vi "配置读取写入.vi"(7 "write":bool, 8 "error in (no error)":errorcluster, 11 "配置":T1={"url"="http://data.watersystem.com.cn:50040", "loginTokenRequest"={"clientId"="wqms_equip", "clientSecret"="2gJxw%vZkRGX8K7Se$^q", "grantType"="password", "password"="123456", "scope"="read", "userName"="equipapi", "userType"="equip"}, "自动获取MN"=TRUE}) -> (0 "error out":errorcluster, 3 "配置输出":T1={"url"="http://dev.watersystem.com.cn:36091", "loginTokenRequest"={"clientId"="test_client", "clientSecret"="test_secret", "grantType"="password", "password"="59315200", "scope"="read", "userName"="STDTEST001", "userType"="equip"}, "自动获取MN"=TRUE})   [LabVIEW 2022 SP3, in "opSignIn.lvlib"]
uses:
  opSignIn.lvlib
  <vilib>/Utility/config.llb/NI_LVConfig.lvlib
  <userlib>/_OpenG.lib/variantconfig/variantconfig.llb/openg_variant_configuration_file.lvlib
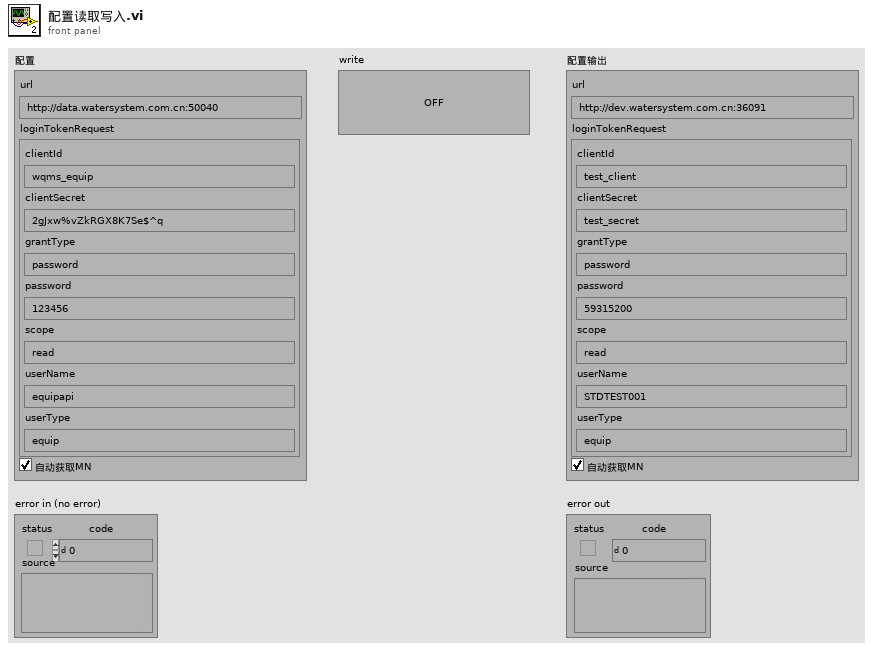
[diagram p1: front panel]
types:
  T1 = cluster{"url":string, "loginTokenRequest":cluster{"clientId":string, "clientSecret":string, "grantType":string, "password":string, "scope":string, "userName":string, "userType":string}, "自动获取MN":bool}
  T2 = typedef "NI_LVConfig.lvlib/Config Data RefNum.ctl" = refnum<k1>
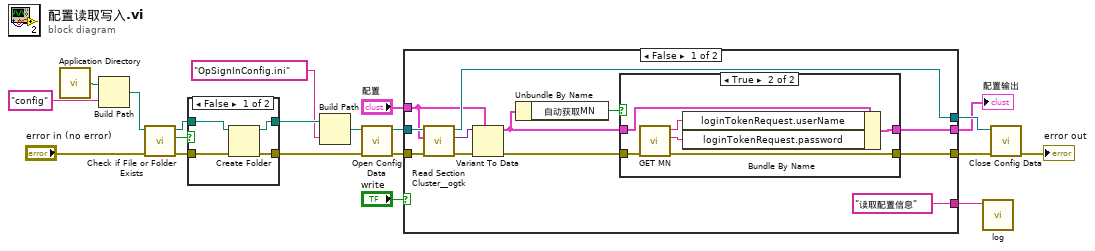
[diagram p0: block diagram]
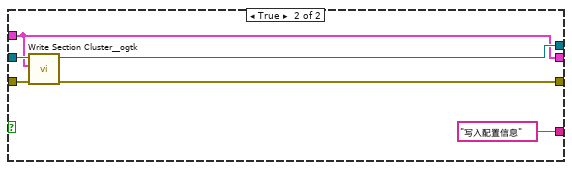
[diagram p3: hidden frame]
diagram:
  n1 = call <vilib>:"Application Directory.vi"() -> ("Application Directory"=w15:path)
  n2 = Build Path(base path=w15, name or relative path="config" ("名称或相对路径")) -> (appended path=w13:path)
  n3 = call <vilib>:"Check if File or Folder Exists.vi"("error in (no error)"="error in (no error)", "path"=w13) -> ("error out"=w10:errorcluster, "file or folder exists?"=w12:bool, "dup path"=w11:path)  [unwired: 7 in]
  n4 = case shown="False" w12 {
    tunnel: w11 -> [w24 w26]
    tunnel: [w23 w26] -> w9
    tunnel: w10 -> [w22 w25]
    tunnel: [w21 w25] -> w3
    frame False {
      n5 = Create Folder(path (use dialog)=w24, error in=w22) -> (created path=w23:path, error out=w21:errorcluster)  [unwired: 1 in, 1 out]
    }
    frame True {
    }
  }
  n6 = Build Path(base path=w9, name or relative path="OpSignInConfig.ini" ("名称或相对路径")) -> (appended path=w8:path)
  n7 = call <vilib>:"Open Config Data.vi"("error in (no error)"=w3, "configuration file path"=w8) -> ("error out"=w18:errorcluster, "refnum"=w20:T2)  [unwired: 7 in, 1 out]
  n8 = case shown="False" "write" {
    tunnel: w20 -> [w38 w52]
    tunnel: "配置" -> [w34 w48]
    tunnel: w18 -> [w37 w51]
    tunnel: [w36 w50] -> w17
    tunnel: [w32 w49] -> w16
    tunnel: [w31 w48] -> w5
    tunnel: ["读取配置信息" "写入配置信息"] -> w1
    frame False {
      n9 = call <userlib>:"Read Section Cluster__ogtk.vi"("error in (no error)"=w37, "Section Formatted Cluster Type"=w34, "refnum"=w38) -> ("error out"=w28:errorcluster, "Section Formatted Cluster"=w35:variant, "dup refnum"=w36:T2)  [unwired: 4 in, 2 out]
      n10 = Variant To Data(error in=w28, type=w34, Variant=w35) -> (data=w30:T1, error out=w27:errorcluster)
      n11 = Unbundle By Name(w30) -> ("自动获取MN"=w29:bool)
      n12 = case shown="True" w29 {
        tunnel: w27 -> [w40 w46]
        tunnel: [w40 w45] -> w32
        tunnel: [w39 w44] -> w31
        tunnel: w30 -> [w39 w41]
        frame False {
        }
        frame True {
          n13 = call "GET MN.vi"("error in (no error)"=w46) -> ("error out"=w45:errorcluster, "PW"=w42:string, "MN"=w43:string)  [unwired: 8 in]
          n14 = Bundle By Name(cluster=w41, "loginTokenRequest.userName"=w43, "loginTokenRequest.password"=w42) -> (w44:T1)
        }
      }
    }
    frame True {
      n15 = call <userlib>:"Write Section Cluster__ogtk.vi"("error in (no error)"=w51, "Section Formatted Cluster"=w48, "refnum"=w52) -> ("error out"=w49:errorcluster, "dup refnum"=w50:T2)  [unwired: 7 in]
    }
  }
  "配置输出" <- w5
  n16 = call "log.vi"("log"=w1) -> ()  [unwired: 11 in]
  n17 = call <vilib>:"Close Config Data.vi"("error in (no error)"=w16, "refnum"=w17) -> ("error out"=→"error out":errorcluster)  [unwired: 8 in, 1 out]
